vi "COM Connect.vi"(6 "VISA resource name":refnum<visa-resource-name>, 7 "Main Front Panel Ref":refnum<vi>, 8 "Error In":errorcluster, 11 "Connection Status":T1=enum."Connected") -> (0 "Error Out":errorcluster, 3 "Connection Status":T1=enum."Connected", 4 "VISA resource name OUT":refnum<visa-resource-name>)   [LabVIEW 2014]
doc: "This VI connects with given com port resource"
uses:
  Controls/Connection Status.ctl
  Controls/Configuration Files.ctl
  Controls/Advanced Connection Settings Cluster.ctl
  <vilib>/Utility/error.llb/DialogType.ctl
  <vilib>/Utility/error.llb/Error Cluster From Error Code.vi
  Convert From XML Configuration Files - Polymorphic/Advanced Connection Settings Polymporhic.vi
  <vilib>/Instr/_visa.llb/VISA Configure Serial Port (Instr).vi
  <vilib>/ErrorRing/Error Ring.xnode
panel:
  # "Connecting..."
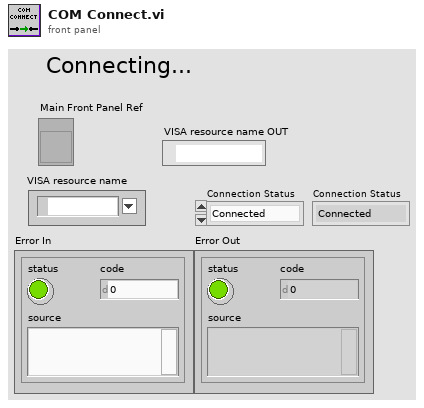
[diagram p1: front panel]
types:
  T1 = typedef "Connection Status.ctl" = enum16{"Disconnected", "Connected"}
  T2 = typedef "Configuration Files.ctl" = string
  T3 = typedef "Advanced Connection Settings Cluster.ctl" = cluster{"Baud Rate":u32, "Data Bits":u16, "Parity":u16, "Stop Bits":u16, "Flow Control":u16, "Termination Char":u8, "Enable Termination Char":bool}
  T4 = typedef "DialogType.ctl" = u16
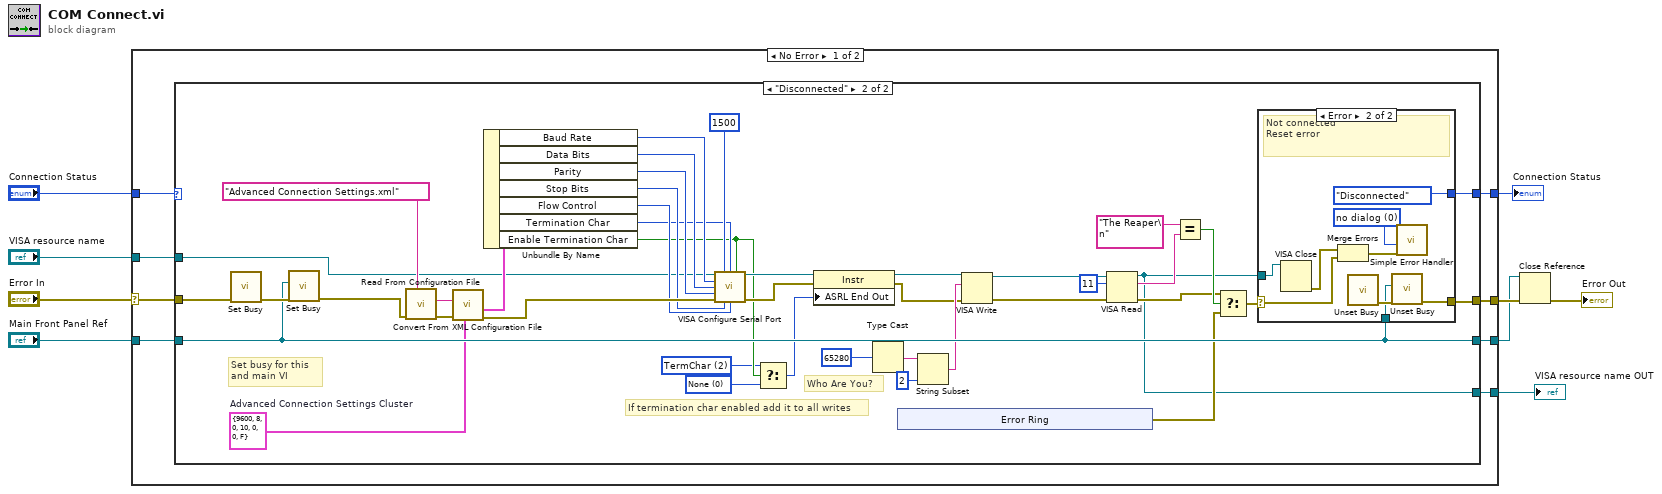
[diagram p0: block diagram]
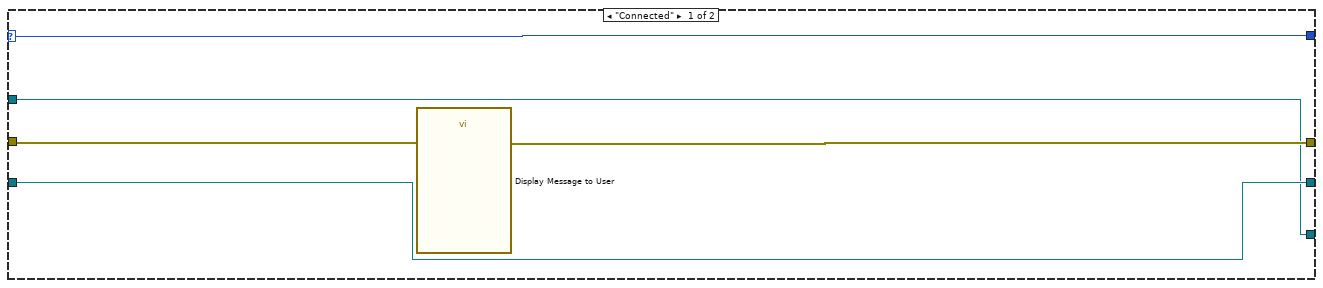
[diagram p2: hidden frame]
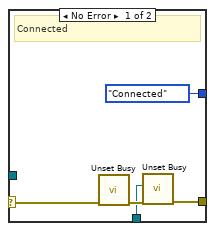
[diagram p3: hidden frame]
diagram:
  n1 = case shown="No Error" "Error In" {
    selector: "Error In" -> [w11 w86]
    tunnel: "Connection Status" -> [w17 w84]
    tunnel: [w16 w86] -> w5
    tunnel: "Main Front Panel Ref" -> [w10 w85]
    tunnel: [w15 w85] -> w4
    tunnel: "VISA resource name" -> [w14 w83]
    tunnel: [w13 w83] -> w2
    tunnel: [w12 w84] -> w1
    frame No Error {
      n2 = case shown="\"Disconnected\"" w17 {
        selector: w17 -> [w20 _]
        tunnel: [w22 w63] -> w16
        tunnel: w10 -> [w21 w62]
        tunnel: [w21 w62] -> w15
        tunnel: w14 -> [w19 w46]
        tunnel: [w19 w26] -> w13
        tunnel: [w20 w48] -> w12
        tunnel: w11 -> [w18 w47]
        frame "Connected" {
          n3 = call "Display Message to User"("error in (no error)"=w18) -> ("error out"=w22:errorcluster)  [unwired: 9 in, 1 out]
        }
        frame "Disconnected" {
          w35 = u16 2 items=["None", "Last Bit", "TermChar", "Break"] ("Serial Settings:End Mode for Writes")
          w37 = u16 0 items=["None", "Last Bit", "TermChar", "Break"] ("Serial Settings:End Mode for Writes")
          w58 = T3 {"Baud Rate"=9600, "Data Bits"=8, "Parity"=0, "Stop Bits"=10, "Flow Control"=0, "Termination Char"=0, "Enable Termination Char"=FALSE}  # Advanced Connection Settings Cluster
          # "Who Are You?"
          # "If termination char enabled add it to all writes"
          # "Set busy for this and main VI"
          n4 = call <vilib>:"Set Busy.vi"("error in (no error)"=w47) -> ("error out"=w64:errorcluster)  [unwired: 9 in, 1 out]
          n5 = call <vilib>:"Set Busy.vi"("error in (no error)"=w64, "VI reference (current VI)"=w62) -> ("error out"=w45:errorcluster)  [unwired: 8 in, 1 out]
          n6 = call "Read From Configuration File.vi"("Settings"=T2 "Advanced Connection Settings.xml", "error in (no error)"=w45) -> ("error out"=w60:errorcluster, "XML Elements"=w59:string)  [unwired: 8 in]
          n7 = call-poly "Convert From XML Configuration File.vi"("Advanced Connection Settings Cluster In"=w58, "error in (no error)"=w60, "XML Elements"=w59) -> ("error out"=w57:errorcluster, "Advanced Connection Settings Cluster Out"=w56:T3)  [unwired: 7 in]
          n8 = Unbundle By Name(w56) -> ("Baud Rate"=w55:u32, "Data Bits"=w54:u16, "Parity"=w53:u16, "Stop Bits"=w51:u16, "Flow Control"=w50:u16, "Termination Char"=w49:u8, "Enable Termination Char"=w38:bool)
          n9 = call-poly "VISA Configure Serial Port"("VISA resource name"=w46, "timeout (10sec)"=u32 1500, "termination char\n(0xA = '\\n' = LF)"=w49, "Enable Termination\nChar (T)"=w38, "baud rate (9600)"=w55, "data bits (8)"=w54, "parity (0:none)"=w53, "error in (no error)"=w57, "stop bits (10: 1 bit)"=w51, "flow control (0:none)"=w50) -> ("VISA resource name out"=w40:refnum<visa-resource-name>, "error out"=w39:errorcluster)  [unwired: 4 in]
          n10 = Select(t=w35, s=w38, f=w37) -> (s? t:f=w36:u16)
          n11 = property class="Instr"(reference=w40, error in=w39, "ASRL End Out"=w36) -> (reference out=w34:refnum<visa-resource-name>, error out=w33:errorcluster)
          n12 = Type Cast(x=65280) -> (*(type *) &x=w43:string)  [unwired: 1 in]
          n13 = xnode "Error Ring"() -> ("error out"=w28:errorcluster)
          n14 = String Subset(string=w43, offset (0)=2) -> (substring=w41:string)  [unwired: 1 in]
          n15 = VISA Write(VISA resource name=w34, write buffer=w41, error in (no error)=w33) -> (VISA resource name out=w25:refnum<visa-resource-name>, error out=w24:errorcluster)  [unwired: 1 out]
          n16 = VISA Read(VISA resource name=w25, byte count=u32 11, error in (no error)=w24) -> (VISA resource name out=w26:refnum<visa-resource-name>, read buffer=w32:string, error out=w29:errorcluster)  [unwired: 1 out]
          n17 = Equal?(x="The Reaper\n", y=w32) -> (x = y?=w30:bool)
          n18 = Select(t=w29, s=w30, f=w28) -> (s? t:f=w27:errorcluster)
          n19 = case shown="Error" w27 {
            selector: w27 -> [w70 w74]
            tunnel: [w73 w81] -> w63
            tunnel: w62 -> [w71 w80]
            tunnel: [Connection_Status."Connected" ("Connection Status") Connection_Status."Disconnected" ("Connection Status")] -> w48
            tunnel: w26 -> [_ w77]
            frame No Error {
              # "Connected"
              n20 = call <vilib>:"Unset Busy.vi"("error in (no error)"=w70) -> ("error out"=w72:errorcluster)  [unwired: 10 in]
              n21 = call <vilib>:"Unset Busy.vi"("error in (no error)"=w72, "VI reference (current VI)"=w71) -> ("error out"=w73:errorcluster)  [unwired: 9 in]
            }
            frame Error {
              w78 = T4 0 items=["no dialog", "OK message", "continue or stop message", "OK message + warnings", "continue/stop + warnings"] ("type of dialog (OK msg:1)")
              # "Not connected\nReset error"
              n22 = VISA Close(VISA resource name=w77) -> (error out=w75:errorcluster)  [unwired: 1 in]
              n23 = Merge Errors(w75, w74) -> (w76:errorcluster)
              n24 = call <vilib>:"Unset Busy.vi"() -> ("error out"=w82:errorcluster)  [unwired: 11 in]
              n25 = call <vilib>:"Unset Busy.vi"("error in (no error)"=w82, "VI reference (current VI)"=w80) -> ("error out"=w81:errorcluster)  [unwired: 9 in]
              n26 = call <vilib>:"Simple Error Handler.vi"("type of dialog (OK msg:1)"=w78, "error in (no error)"=w76) -> ()  [unwired: 3 in, 5 out]
            }
          }
        }
      }
    }
    frame Error {
    }
  }
  "Connection Status" <- w1
  "VISA resource name OUT" <- w2
  n27 = Close Reference(reference=w4, error in (no error)=w5) -> (error out=→"Error Out":errorcluster)
